vi "FinalizeDependencyListGeneration.vi"(8 "error in (no error)":errorcluster, 11 "CDependencyInspector in":refnum<class "CDependencyInspection.lvclass">) -> (0 "error out":errorcluster, 3 "CDependencyInspector out":refnum<class "CDependencyInspection.lvclass">)   [LabVIEW 2020, in "DependencyInspection.lvlib" / "CDependencyInspection.lvclass"]
uses:
  CDependencyInspection.lvclass
  CDependencyList/CDependencyList.lvclass
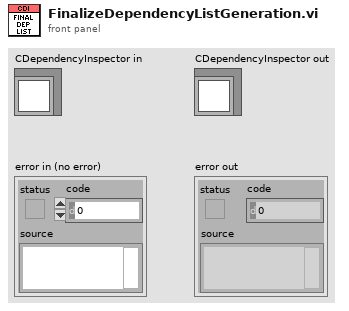
[diagram p1: front panel]
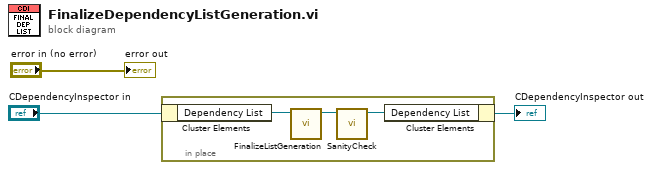
[diagram p0: block diagram]
diagram:
  n1 = in-place {
    n2 = in-place-cluster #1("CDependencyInspector in") -> ("Dependency List"=w5:refnum<class "CDependencyList.lvclass">)
    n3 = call-dynamic "FinalizeListGeneration.vi"("CDependencyList in"=w5) -> ("CDependencyList out"=w4:refnum<class "CDependencyList.lvclass">)  [unwired: 9 in, 1 out]
    n4 = call-dynamic "SanityCheck.vi"("CDependencyList in"=w4) -> ("CDependencyList out"=w6:refnum<class "CDependencyList.lvclass">)  [unwired: 8 in, 2 out]
    n5 = in-place-cluster #1("Dependency List"=w6) -> (→"CDependencyInspector out":refnum<class "CDependencyInspection.lvclass">)
  }
  "error out" <- "error in (no error)"
